vi "InsertMenuItemsWithShortcut.vi"(6 "Insert After (last)":i32, 8 "error in (no error)":errorcluster, 9 "Sub Items":T1(array[cluster]), 10 "Target Tag":string, 11 "menu ref":refnum<k9>) -> (0 "error out":errorcluster, 1 "Sub Item Tags":string[](array[string]), 3 "menu ref out":refnum<k9>, 4 "Sub Item Names":string[](array[string]))   [LabVIEW 2020]
uses:
  <vilib>/Utility/miscctls.llb/LVMenuShortCut.ctl
panel:
  # "セパレータは APP_SEPARATOR"
  # "先頭に置くには -1\n2番目に入れるなら 0\n大きすぎれば末尾"
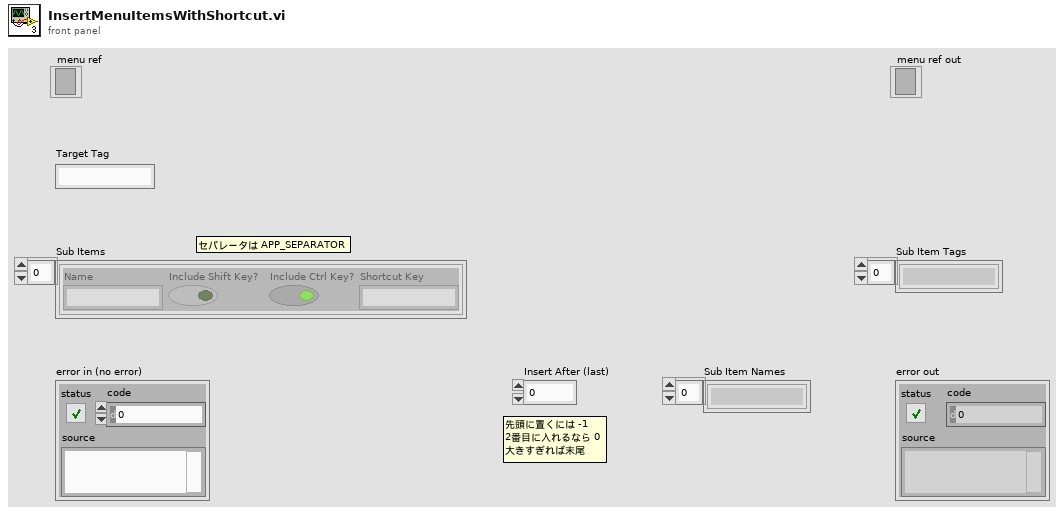
[diagram p1: front panel]
types:
  T1 = cluster{"Name":string, "Include Shift Key?":bool, "Include Ctrl Key?":bool, "Shortcut Key":string}[]
  T2 = typedef "LVMenuShortCut.ctl" = cluster{"Include Shift Key?":bool, "Include Ctrl Key?":bool, "Shortcut Key":string}
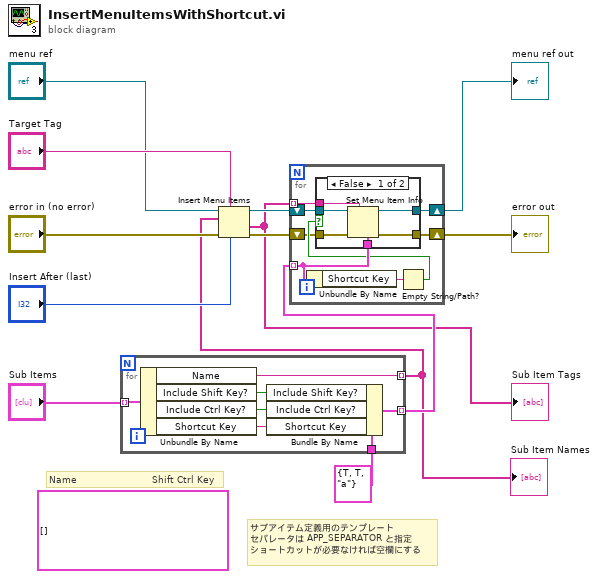
[diagram p0: block diagram]
diagram:
  (unwired) T1 [] ("Menu Short Cut")
  # "Name                         Shift Ctrl Key"
  # "サブアイテム定義用のテンプレート\nセパレータは APP_SEPARATOR と指定\nショートカットが必要なければ空欄にする"
  n1 = for {
    tunnel: "Sub Items" -> [w20] mode=indexing
    tunnel: [w19] -> w1 mode=indexing
    tunnel: [w15] -> w11 mode=indexing
    tunnel: T2 {"Include Shift Key?"=TRUE, "Include Ctrl Key?"=TRUE, "Shortcut Key"="a"} ("Menu Short Cut") -> [w14]
    n2 = Unbundle By Name(w20) -> ("Name"=w19:string, "Include Shift Key?"=w18:bool, "Include Ctrl Key?"=w17:bool, "Shortcut Key"=w16:string)
    n3 = Bundle By Name(cluster=w14, "Include Shift Key?"=w18, "Include Ctrl Key?"=w17, "Shortcut Key"=w16) -> (w15:T2)
  }
  "Sub Item Names" <- w1
  n4 = Insert Menu Items(4:"Insert After (last)", 5:"Target Tag", 6:"error in (no error)", 8:w1, 9:"menu ref") -> (0:w10:errorcluster, 1:w3:string[], 3:w12:refnum<k9>)  [unwired: 1 in]
  "Sub Item Tags" <- w3
  n5 = for {
    tunnel: w3 -> [w28] mode=indexing
    tunnel: w11 -> [w27] mode=indexing
    shift-right: [w23] -> w9
    shift-left: w12 -> [w24]
    shift-right: [w21] -> w8
    shift-left: w10 -> [w22]
    n6 = Unbundle By Name(w27) -> ("Shortcut Key"=w26:string)
    n7 = Empty String/Path?(string/path=w26) -> (empty?=w25:bool)
    n8 = case shown="False" w25 {
      tunnel: w28 -> [w34 _]
      tunnel: w27 -> [w33 _]
      tunnel: w24 -> [w32 w36]
      tunnel: [w31 w36] -> w23
      tunnel: w22 -> [w30 w35]
      tunnel: [w29 w35] -> w21
      frame False {
        n9 = Set Menu Item Info(4:w33, 7:w34, 8:w30, 11:w32) -> (0:w29:errorcluster, 3:w31:refnum<k9>)  [unwired: 3 in]
      }
      frame True {
      }
    }
  }
  "menu ref out" <- w9
  "error out" <- w8
